vi "changeIntegrationTime.vi"(8 "error in (no error)":errorcluster, 10 "ElectrometerController in":refnum<class "ElectrometerController.lvclass">, 11 "ElectrometerState in":refnum<class "ElectrometerState.lvclass">) -> (0 "error out":errorcluster, 2 "ElectrometerController out":refnum<class "ElectrometerController.lvclass">, 3 "ElectrometerState out":refnum<class "ElectrometerState.lvclass">)   [LabVIEW 2016, in "ElectrometerState.lvclass"]
uses:
  ElectrometerState.lvclass
  ElectrometerController/ElectrometerController.lvclass
  ts_electrometeruserevents/Typedefs/RejectedCommand.ctl
  ts_electrometeruserevents/Typedefs/CommandValue.ctl
  ts_electrometeruserevents/Typedefs/StateValue.ctl
  ts_electrometeruserevents/Typedefs/ElectrometerTypedefs.lvlib
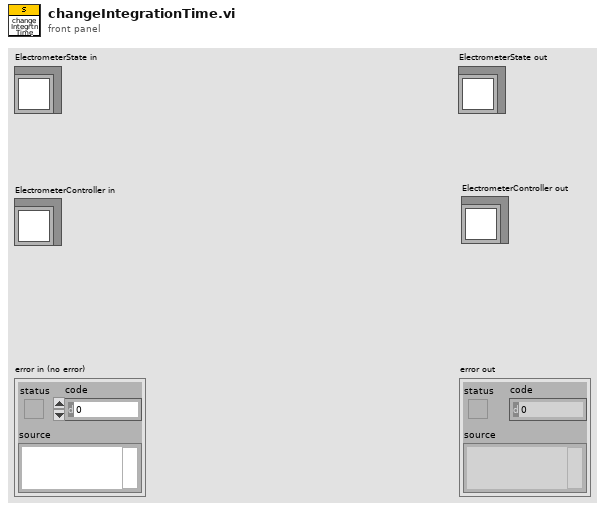
[diagram p1: front panel]
types:
  T1 = typedef "ElectrometerTypedefs.lvlib/RejectedCommand.ctl" = cluster{"CommandValue":T2, "StateValue":T3, "Time Stamp":dbl}
  T2 = typedef "ElectrometerTypedefs.lvlib/CommandValue.ctl" = enum16{"ClearError", "Disable", "Enable", "Exit", "GoToStandby", "OnHeartbeat", "OnIncomingMessagingError", "OnInterrupt", "Start", "SetDigitalFilter", "StartScan", "StartScanDt", "StartScanReachIntensity", "StopScan", "SetIntegrationTime", "PerformZeroCalib", "SetRange", "SetMode", "Power"}
  T3 = typedef "ElectrometerTypedefs.lvlib/StateValue.ctl" = enum16{"OffState", "StandbyState", "DisabledState", "EnabledState", "FaultState", "SetDurationReadingState", "ConfiguringState", "ReadyState", "ManualReadingState", "UntilIntentisyReadingState"}
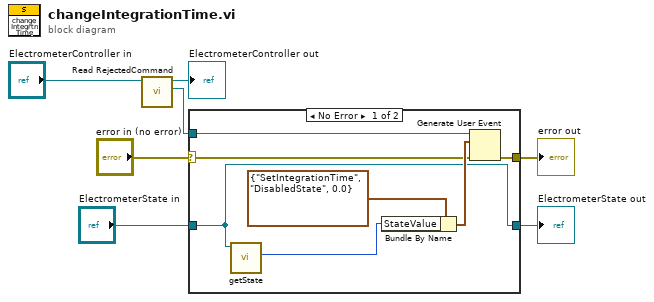
[diagram p0: block diagram]
diagram:
  n1 = call-dynamic "Read RejectedCommand.vi"("ElectrometerController in"="ElectrometerController in") -> ("RejectedCommand"=w1:refnum<user-event>, "ElectrometerController out"=→"ElectrometerController out":refnum<class "ElectrometerController.lvclass">)  [unwired: 8 in, 1 out]
  n2 = case shown="No Error" "error in (no error)" {
    selector: "error in (no error)" -> [w11 w16]
    tunnel: [w10 w16] -> w6
    tunnel: [w9 w15] -> w4
    tunnel: "ElectrometerState in" -> [w9 w15]
    tunnel: w1 -> [w8 _]
    frame No Error {
      n3 = call-dynamic "getState.vi"("State in"=w9) -> ("StateValue"=w12:T3)  [unwired: 8 in, 2 out]
      n4 = Bundle By Name(cluster=T1 {"CommandValue"=enum."SetIntegrationTime", "StateValue"=enum."DisabledState", "Time Stamp"=0.0} ("event data"), "StateValue"=w12) -> (w13:T1)
      n5 = Generate User Event(user event=w8, event data cluster=w13, error in=w11) -> (error out=w10:errorcluster)  [unwired: 1 in, 1 out]
    }
    frame Error {
    }
  }
  "error out" <- w6
  "ElectrometerState out" <- w4
